vi "GetSessionAction.vi"(8 "error in (no error)":errorcluster, 11 "Refnum in":refnum<k20>) -> (0 "error out":errorcluster, 1 "ActionValue":string[](array[string]), 2 "ActionName":string[](array[string]), 3 "node out":refnum<k20>)   [LabVIEW 2015]
uses:
  <vilib>/xml/Close Reference(Node).vi
  <vilib>/xml/NI_XML.lvlib
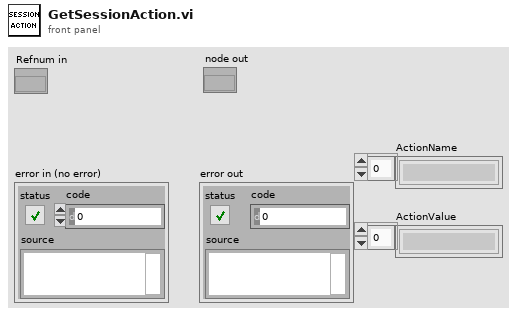
[diagram p1: front panel]
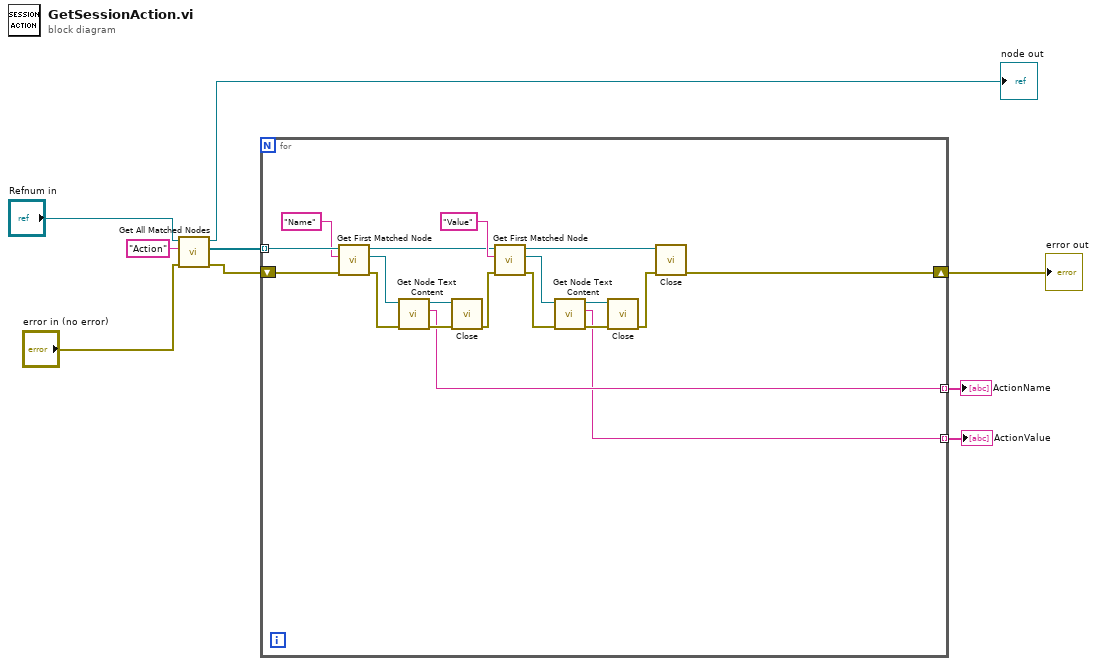
[diagram p0: block diagram]
diagram:
  n1 = call <vilib>:"Get All Matched Nodes.vi"("error in (no error)"="error in (no error)", "XPath expression"="Action", "node in"="Refnum in") -> ("error out"=w4:errorcluster, "node result array"=w5:refnum<k20>[], "node out"=→"node out":refnum<k20>)  [unwired: 6 in]
  n2 = for {
    tunnel: w5 -> [w28] mode=indexing
    shift-right: [w12] -> w3
    shift-left: w4 -> [w26]
    tunnel: [w11] -> w2 mode=indexing
    tunnel: [w10] -> w1 mode=indexing
    n3 = call <vilib>:"Get First Matched Node.vi"("error in (no error)"=w26, "XPath expression"="Name", "node in"=w28) -> ("error out"=w22:errorcluster, "node result"=w25:refnum<k20>, "node out"=w15:refnum<k20>)  [unwired: 6 in]
    n4 = call <vilib>:"Get Node Text Content.vi"("error in (no error)"=w22, "node in"=w25) -> ("error out"=w23:errorcluster, "node text"=w11:string, "node out"=w24:refnum<k20>)  [unwired: 7 in]
    n5 = call-poly <vilib>:"Close.vi"("error in (no error)"=w23, "node"=w24) -> ("error out"=w16:errorcluster)  [unwired: 7 in]
    n6 = call <vilib>:"Get First Matched Node.vi"("error in (no error)"=w16, "XPath expression"="Value", "node in"=w15) -> ("error out"=w21:errorcluster, "node result"=w18:refnum<k20>, "node out"=w14:refnum<k20>)  [unwired: 6 in]
    n7 = call <vilib>:"Get Node Text Content.vi"("error in (no error)"=w21, "node in"=w18) -> ("error out"=w20:errorcluster, "node text"=w10:string, "node out"=w19:refnum<k20>)  [unwired: 7 in]
    n8 = call-poly <vilib>:"Close.vi"("error in (no error)"=w20, "node"=w19) -> ("error out"=w13:errorcluster)  [unwired: 7 in]
    n9 = call-poly <vilib>:"Close.vi"("error in (no error)"=w13, "node"=w14) -> ("error out"=w12:errorcluster)  [unwired: 7 in]
  }
  "error out" <- w3
  "ActionName" <- w2
  "ActionValue" <- w1
